vi "getTaskReference.vi"(8 "error in (no error)":errorcluster, 11 "TaskMock in":refnum<class "TaskMock.lvclass">) -> (0 "error out":errorcluster, 2 "taskRef":refnum<vi>, 3 "TaskMock out":refnum<class "TaskMock.lvclass">)   [LabVIEW 2023, in "TaskMock.lvclass"]
uses:
  TaskMock.lvclass
  task.vi
  TaskMock.lvclass/TaskMock.ctl
  brokenTask.vi
  taskWithWrongConnectorPane.vi
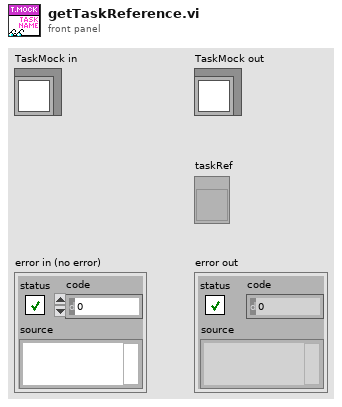
[diagram p1: front panel]
types:
  T1 = enum16{"ValidTask", "BrokenTask", "InvalidConnectorPaneTask"}
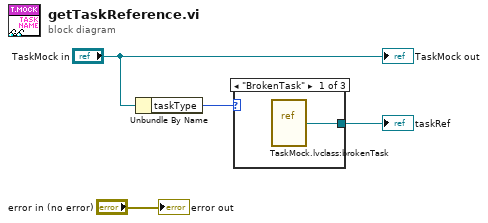
[diagram p0: block diagram]
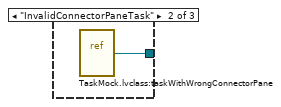
[diagram p2: hidden frame]
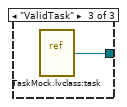
[diagram p3: hidden frame]
diagram:
  n1 = Unbundle By Name("TaskMock in") -> ("taskType"=w1:T1)
  n2 = case shown="\"BrokenTask\"" w1 {
    tunnel: [w5 w6 w7] -> w3
    frame "BrokenTask" {
      n3 = vi-ref "TaskMock.lvclass:brokenTask.vi"() -> (w5:refnum<vi>)
    }
    frame "InvalidConnectorPaneTask" {
      n4 = vi-ref "TaskMock.lvclass:taskWithWrongConnectorPane.vi"() -> (w6:refnum<vi>)
    }
    frame "ValidTask" {
      n5 = vi-ref "TaskMock.lvclass:task.vi"() -> (w7:refnum<vi>)
    }
  }
  "taskRef" <- w3
  "error out" <- "error in (no error)"
  "TaskMock out" <- "TaskMock in"
